vi "测验程序3.vi"() -> ()   [LabVIEW 2017]
uses:
  <vilib>/userdefined/High Color/IMAQdx.ctl
  <vilib>/Platform/TimedLoop/XDataNode/timing_clust.ctl
  <vilib>/Platform/TimedLoop/XDataNode/nitl_modes.ctl
  <vilib>/Platform/TimedLoop/XDataNode/wakeup.ctl
  <vilib>/myRIO/Common/Instrument Driver Framework/myRIO v1.0/UART/vis/myRIO v1.0 Close UART.vi
  <vilib>/FPGAPlugInAG/myRIO-1900/niLvFpga_Open_myRIO-1900.vi
  <vilib>/rvi/interface/common/dynamic/niFpgaDynamicAddResources.vi
  <vilib>/myRIO/Common/Instrument Driver Framework/Utilities/vis/FPGA Ref Manager.vi
  <vilib>/Utility/error.llb/Error Cluster From Error Code.vi
  <vilib>/myRIO/Common/Instrument Driver Framework/Utilities/vis/Ref Counter.vi
  <vilib>/rvi/errors/niLvFpgaAdjustHostInterfaceError.vi
  <vilib>/FPGAPlugInAG/Dynamic/niLvFpga_Close_Dynamic.vi
  <vilib>/myRIO/Common/Instrument Driver Framework/myRIO v1.0/myRIO v1.0 Reset FPGA.vi
  <vilib>/myRIO/Common/Instrument Driver Framework/myRIO v1.0/IRQ/vis/myRIO v1.0 IRQ Info FGV.vi
  <vilib>/myRIO/Common/Instrument Driver Framework/myRIO v1.0/IRQ/vis/myRIO v1.0 Timer IRQ Info FGV.vi
  <vilib>/myRIO/Common/Instrument Driver Framework/myRIO v1.0/IRQ/vis/myRIO v1.0 ISR Agent.vi
  <vilib>/Platform/TimedLoop/XDataNode/XDataNode.xnode
  <vilib>/rvi/interface/nirviOpenFPGA/nirviOpenFPGA.xnode
  <vilib>/rvi/interface/nirviReadWriteControl/nirviReadWriteControl.xnode
  <vilib>/rvi/interface/nirviCloseFPGA/nirviCloseFPGA.xnode
  <vilib>/Platform/TimedLoop/XDataNode/XDNodeRunTimeDep.lvlib
  <vilib>/myRIO/Instrument Drivers/Utilities/Utilities.lvlib
  NiFpgaLv.dll
  <vilib>/rvi/interface/Simulation/niFpgaSimulationCallBeginRW.vi
  <vilib>/vision/driver/NI_Vision_Acquisition_Software.lvlib
  <vilib>/vision/NI_Vision_Development_Module.lvlib
panel:
  out "货物类型":u32
  in  "Reset":bool
  in  "Reset to gait 0":bool
  in  "停止":bool
  out "数量":i32[](array[numeric])
  in  "保留图像？":bool
  in  "停止 2":bool
  in  "初始步态":u16
  in  "开始":bool
  out "QTI":bool
  out "当前步态":u16
  out "超声波":u32[](array[numeric])
  # "4小蓝"
  # "3小红"
  # "2大蓝"
  # "100000"
  # "1大红"
  # "70000"
  # "0异常"
  # "25000"
  # "14600夹取高度"
  # "700夹住"
  # "-1010"
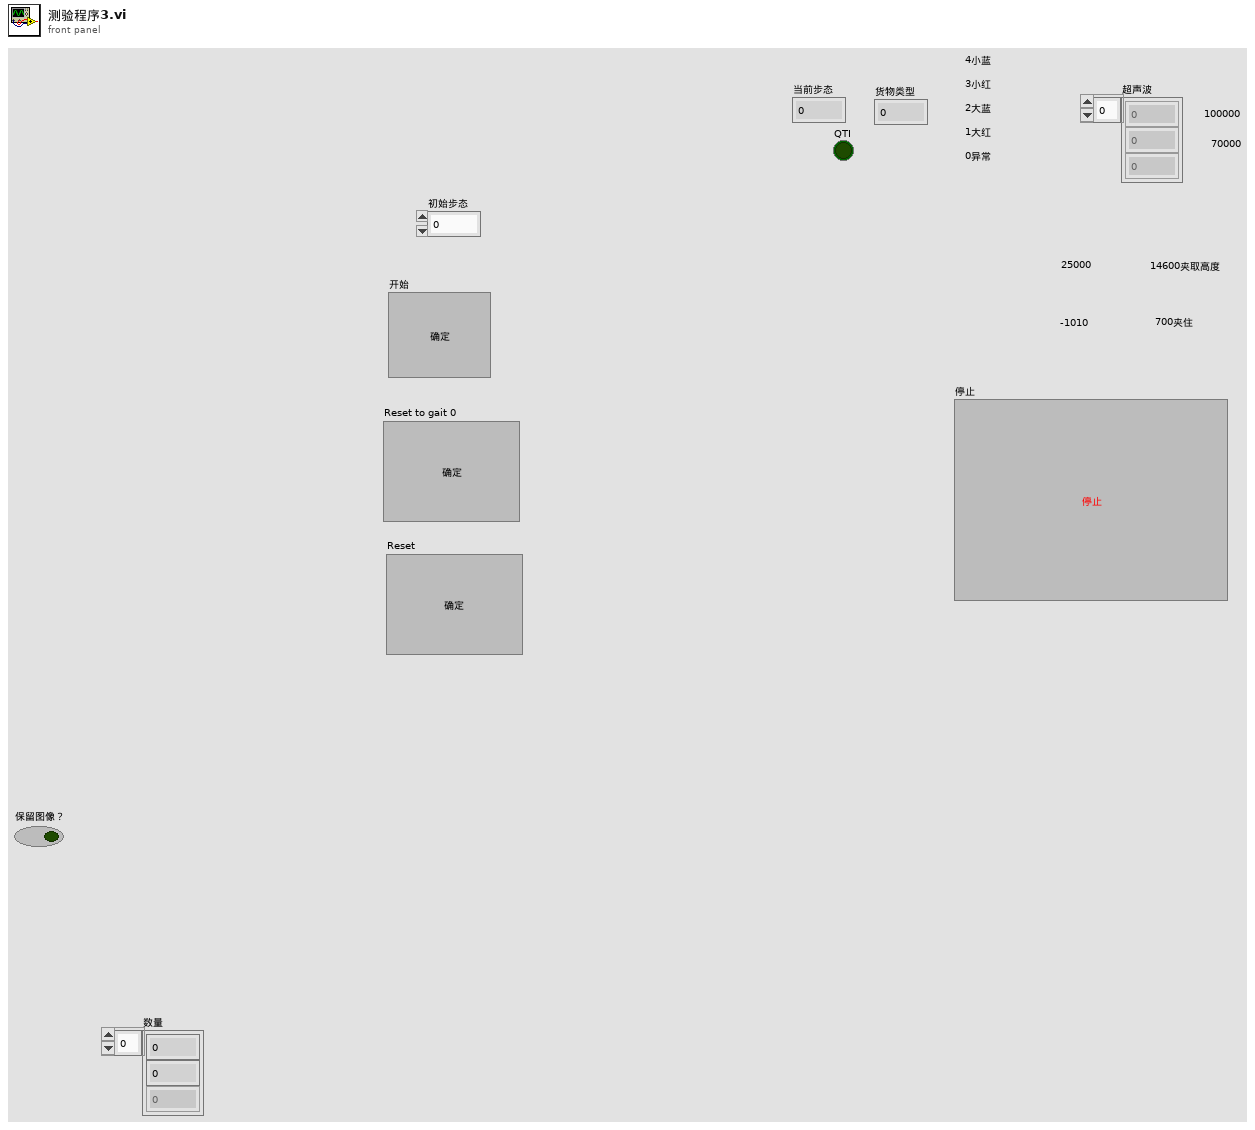
[diagram p1: front panel]
types:
  T1 = typedef "IMAQdx.ctl" = refnum<k21>
  T2 = typedef "IMAQ Image.ctl" = refnum<image>
  T3 = typedef "XDNodeRunTimeDep.lvlib/timing_clust.ctl" = cluster{"Expected End [f-1]":u64, "Actual End [f-1]":u64, "Finished Late? [f-1]":bool, "Expected End [i-1]":u64, "Actual End [i-1]":u64, "Finished Late? [i-1]":bool, "Expected Start [i]":u64, "Actual Start [i]":u64, "Expected Start [f]":u64, "Actual Start [f]":u64, "Source Name":string, "Structure Name":string, "Period":i64, "Deadline":i64, "Offset":i64, "Start":i64, "Priority":i32, "Timeout":i32, "Mode":T4, "Wakeup Reason":T5, "Error":errorcluster, "Source Type":string, "Secondary Source Type":string, "Global End Time":u64, "Global Start Time":u64, "Frame Duration":u64, "Iteration Duration":u64, "Assigned CPU":i32, "I/O Scan Engine Mode":u32}
  T4 = typedef "XDNodeRunTimeDep.lvlib/nitl_modes.ctl" = enum32{"No Change", "Process missed periods, maintain original phase", "Discard missed periods, maintain original phase", "Process missed periods, ignore original phase", "Discard missed periods, ignore original phase"}
  T5 = typedef "XDNodeRunTimeDep.lvlib/wakeup.ctl" = enum32{"Normal", "Aborted", "Asynchronous wakeup", "Timing source error", "Timed loop error", "Timeout"}
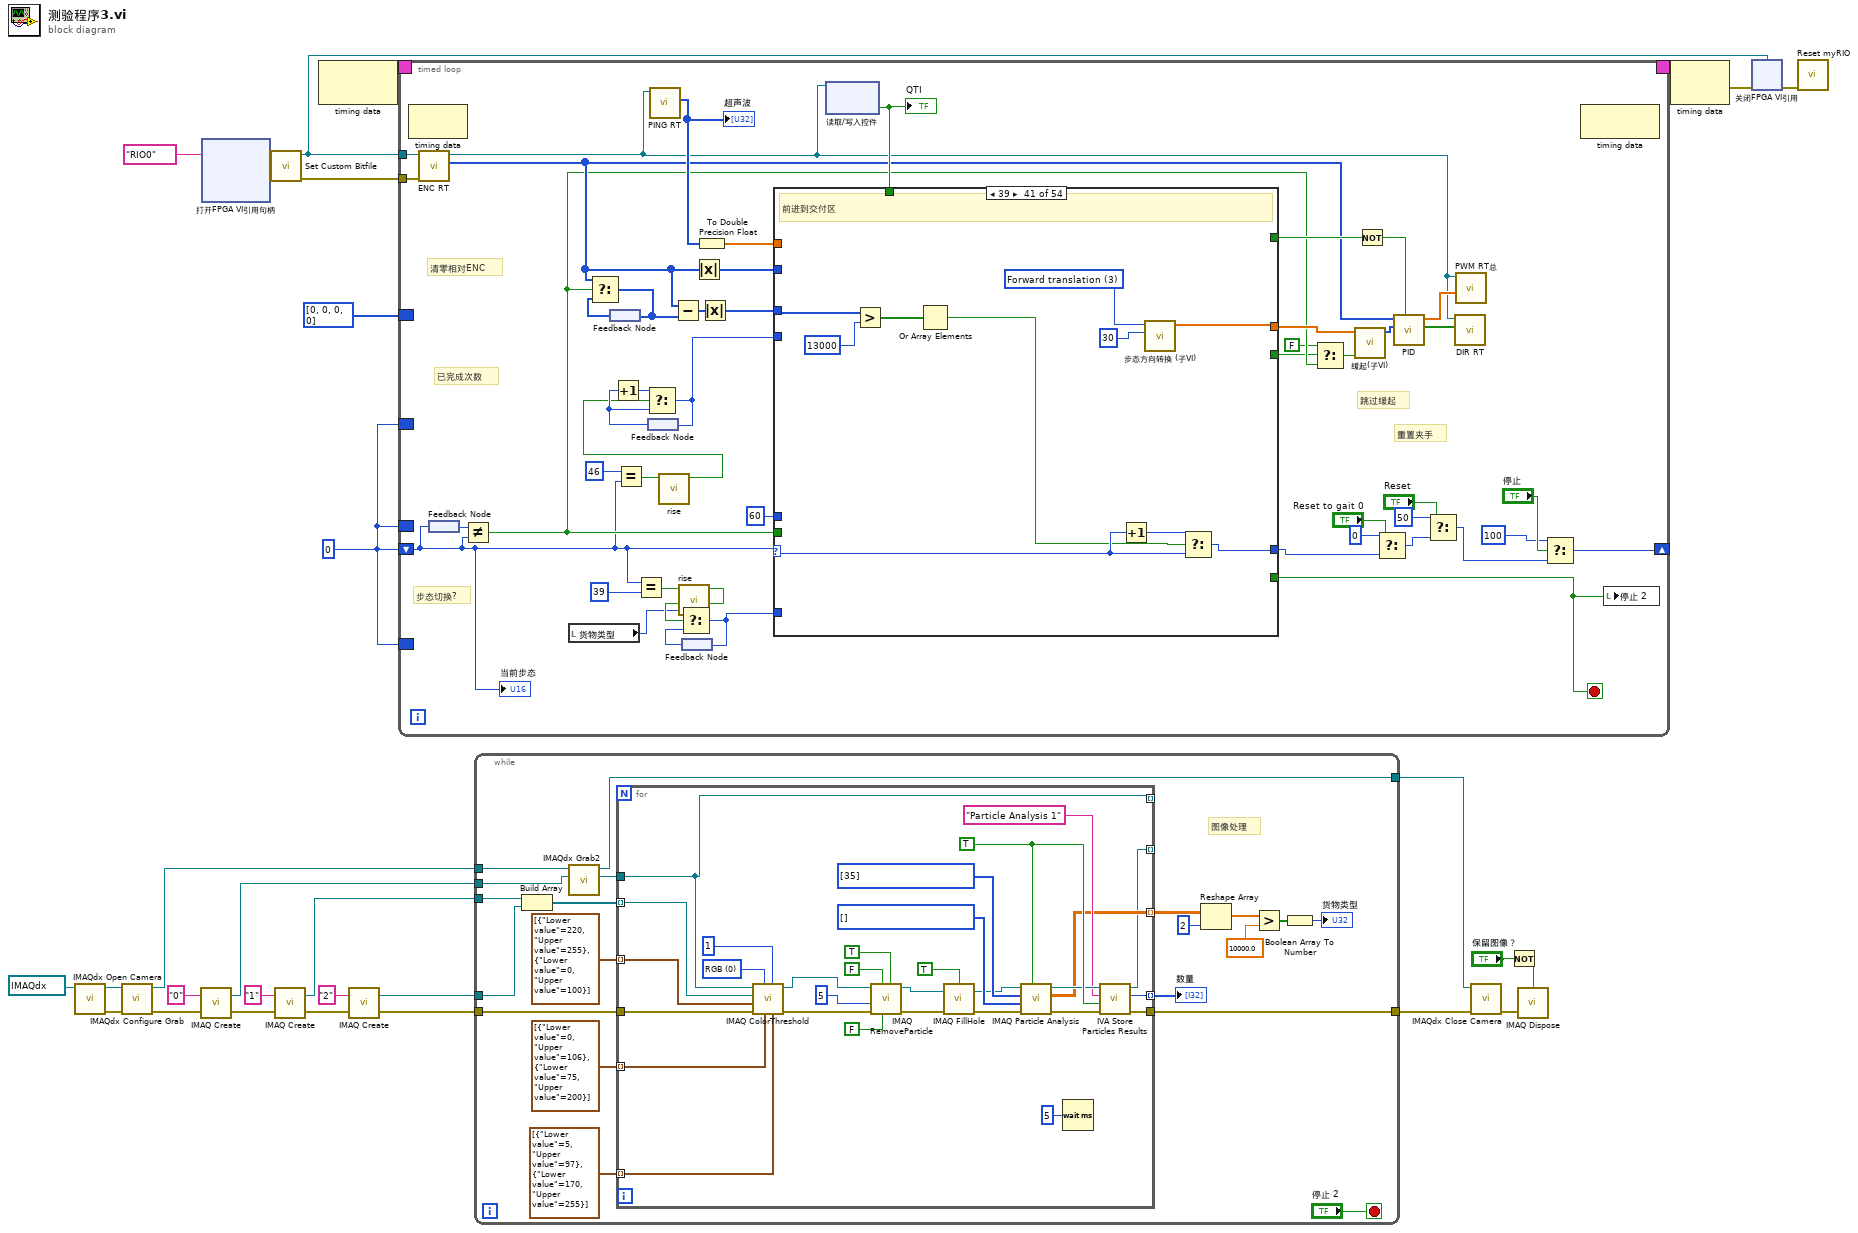
[diagram p0: block diagram]
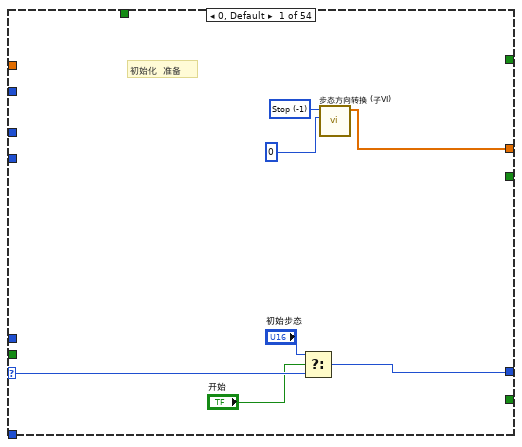
[diagram p2: hidden frame]
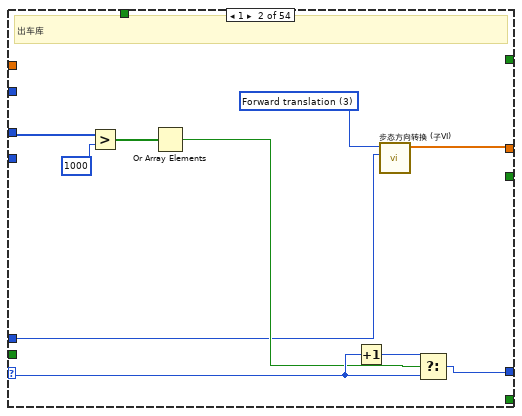
[diagram p3: hidden frame]
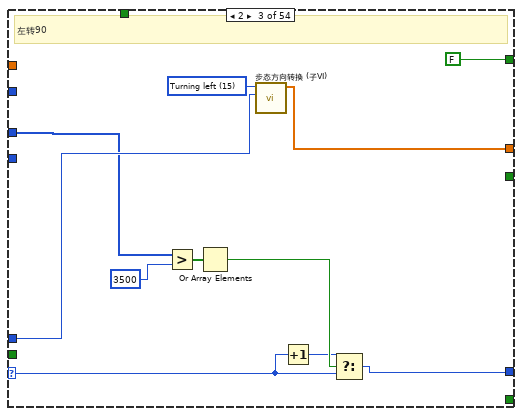
[diagram p4: hidden frame]
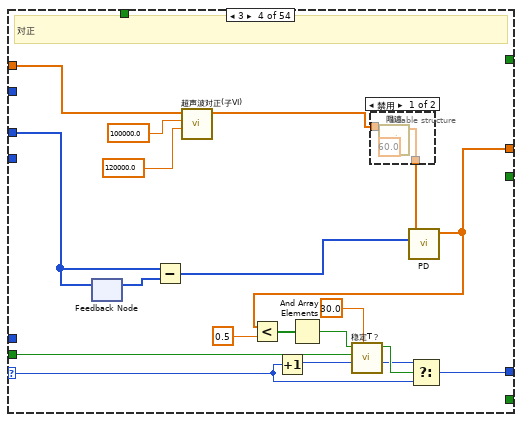
[diagram p5: hidden frame]
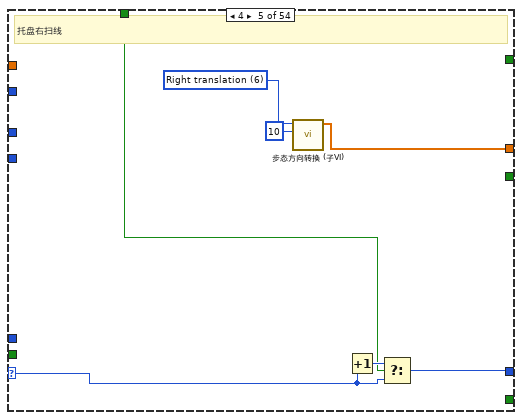
[diagram p7: hidden frame]
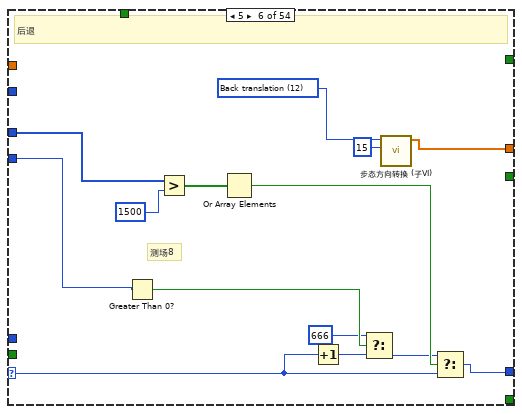
[diagram p8: hidden frame]
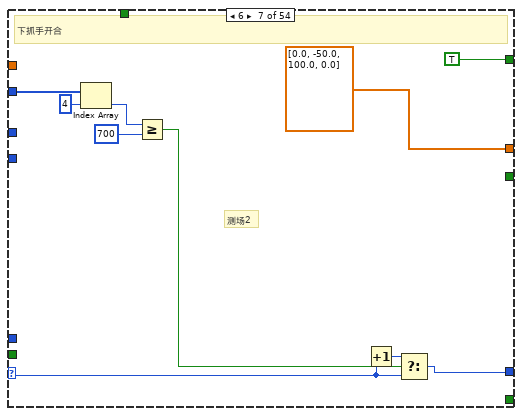
[diagram p9: hidden frame]
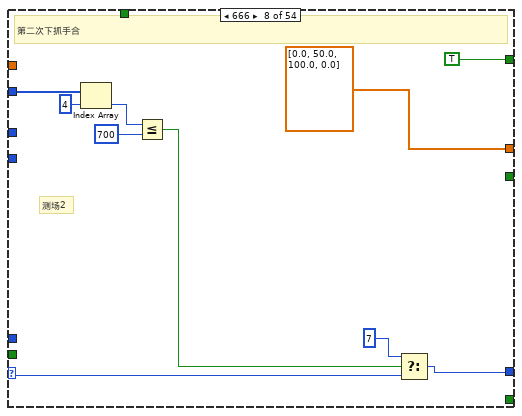
[diagram p10: hidden frame]
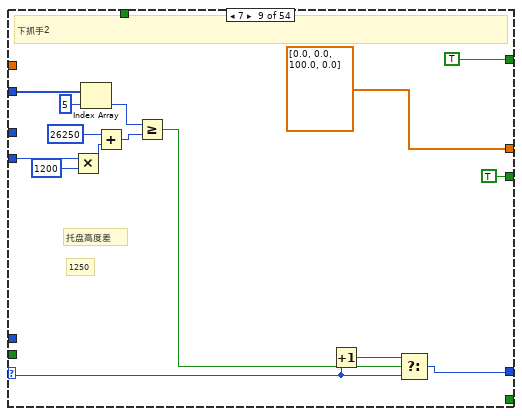
[diagram p11: hidden frame]
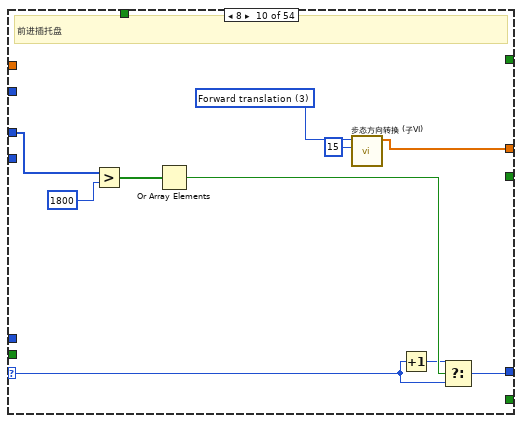
[diagram p12: hidden frame]
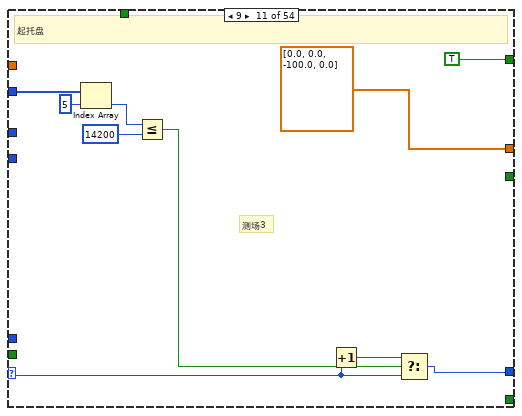
[diagram p13: hidden frame]
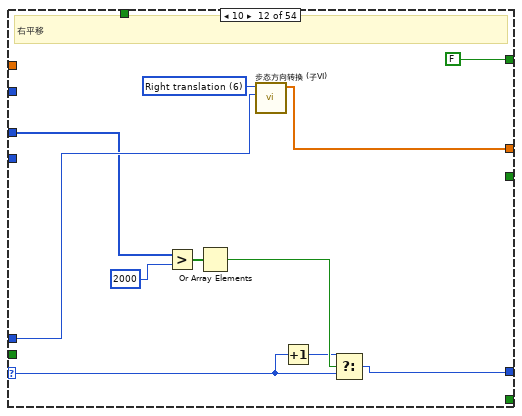
[diagram p14: hidden frame]
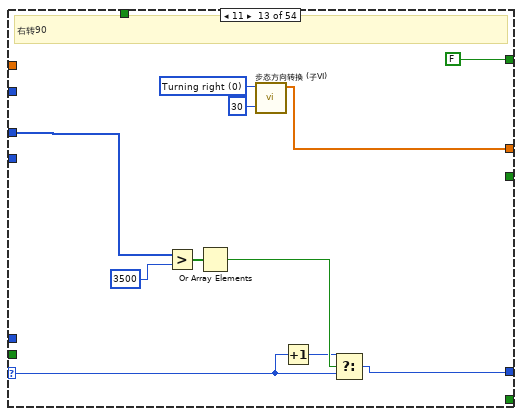
[diagram p15: hidden frame]
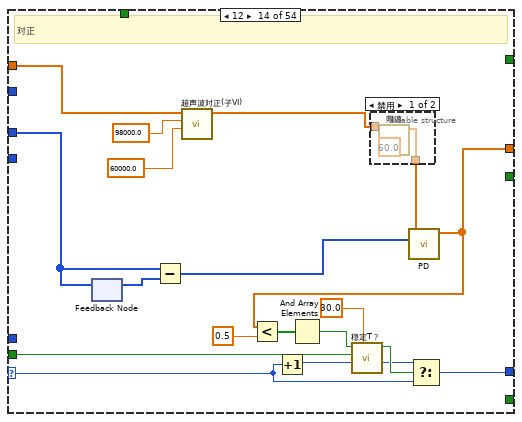
[diagram p16: hidden frame]
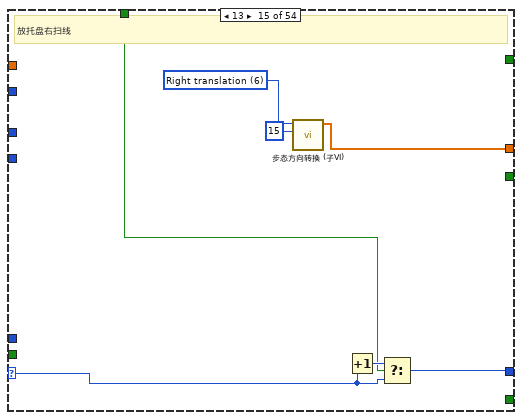
[diagram p18: hidden frame]
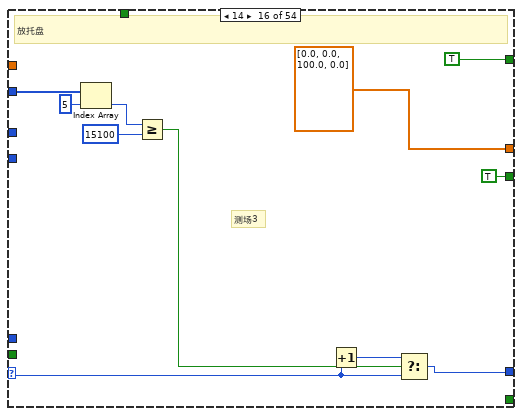
[diagram p19: hidden frame]
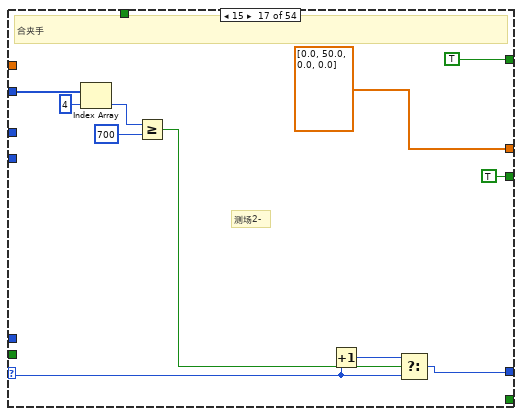
[diagram p20: hidden frame]
diagram:
  w1 = u16 0 ("初始步态")
  n1 = call <vilib>:"IMAQdx Open Camera.vi"("Session In"=T1 "cam0") -> ("error out"=w16:errorcluster, "Session Out"=w15:T1)  [unwired: 9 in]
  n2 = call <vilib>:"IMAQdx Configure Grab.vi"("error in"=w16, "Session In"=w15) -> ("error out"=w13:errorcluster, "Session Out"=w20:T1)  [unwired: 8 in]
  n3 = call "IMAQ Create"("Image Name"="0", "error in (no error)"=w13) -> ("New Image"=w18:T2, "error out"=w11:errorcluster)  [unwired: 3 in]
  n4 = xnode "打开FPGA VI引用句柄"("资源名称"=tag "RIO0") -> ("FPGA VI引用输出"=w25:refnum<k20>, "错误输出"=w24:errorcluster)  [unwired: 1 in]
  n5 = call <vilib>:"Set Custom Bitfile.vi"("error in (no error)"=w24, "Custom FPGA Reference In"=w25) -> ("error out"=w23:errorcluster, "Custom FPGA Reference Out"=w21:refnum<k20>)  [unwired: 8 in]
  n6 = call "IMAQ Create"("Image Name"="1", "error in (no error)"=w11) -> ("New Image"=w8:T2, "error out"=w9:errorcluster)  [unwired: 3 in]
  n7 = node-c288() -> (w30:T3)  [unwired: 1 in]
  n8 = call "IMAQ Create"("Image Name"="2", "error in (no error)"=w9) -> ("New Image"=w7:T2, "error out"=w6:errorcluster)  [unwired: 3 in]
  n9 = timed-loop {
    timing: w30 -> [_]
    timing-out: [_] -> w29
    shift-right: [w58] -> _
    shift-left: w1 -> [w33]
    border: w1 -> [_]
    border: i32[] [0, 0, 0, 0] ("ENC") -> [_]
    tunnel: w23 -> [w75]
    tunnel: w21 -> [w72]
    border: w1 -> [_]
    border: w1 -> [_]
    stop <- w44 stop-if-true
    # "已完成次数"
    # "重置夹手"
    # "跳过缓起"
    # "步态切换?"
    # "清零相对ENC"
    n10 = node-c288() -> ()  [unwired: 1 in, 1 out]
    n11 = call "ENC RT.vi"("错误输入（无错误）"=w75, "Custom FPGA Reference Out"=w72) -> ("ENC"=w62:i32[], "FPGA VI引用输出"=w60:refnum<k20>)  [unwired: 7 in, 1 out]
    n12 = feedback-in #1(w33) -> ()
    n13 = feedback #1() -> (w76:u16)
    n14 = Not Equal?(x=w76, y=w33) -> (x != y?=w52:bool)
    n15 = local read "货物类型"() -> (w32:u32)
    n16 = feedback #2() -> (w74:i32[])
    n17 = Select(t=w62, s=w52, f=w74) -> (s? t:f=w59:i32[])
    n18 = feedback-in #2(w59) -> ()
    n19 = Equal?(x=u16 46 ("y"), y=w33) -> (x = y?=w39:bool)
    n20 = Equal?(x=w33, y=u16 39) -> (x = y?=w36:bool)
    n21 = feedback #3() -> (w42:u16)
    n22 = Increment(x=w42) -> (x+1=w41:u16)
    n23 = call "PING RT.vi"("引用句柄输入"=w60) -> ("PING"=w66:u32[])  [unwired: 8 in, 2 out]
    "超声波" <- w66
    n24 = call "rise.vi"("TF"=w39) -> ("UP?"=w38:bool)  [unwired: 10 in]
    n25 = Select(t=w41, s=w38, f=w42) -> (s? t:f=w40:u16)
    n26 = feedback-in #3(w40) -> ()
    n27 = Subtract(x=w62, y=w59) -> (x-y=w67:i32[])
    n28 = call "rise.vi"("TF"=w36) -> ("UP?"=w37:bool)  [unwired: 10 in]
    n29 = feedback #4() -> (w35:u32)
    n30 = Select(t=w32, s=w37, f=w35) -> (s? t:f=w31:u32)
    n31 = feedback-in #4(w31) -> ()
    n32 = Absolute Value(x=w62) -> (abs(x)=w61:i32[])
    n33 = To Double Precision Float(number=w66) -> (double precision float=w65:dbl[])
    n34 = Absolute Value(x=w67) -> (abs(x)=w63:i32[])
    n35 = xnode "读取/写入控件"("FPGA VI引用输入"=w60) -> ("QTI"=w64:bool)  [unwired: 1 in, 2 out]
    "QTI" <- w64
    n36 = case shown="39" w33 {
      selector: w33 -> [w84 w88 w99 w122 w132 w145 w156 w167 w182 w186 w202 w208 w220 w242 w252 w264 w275 w279 w292 w325 w336 w347 w354 w378 w384 w395 w405 w415 w421 w455 w461 w469 w491 w497 w508 w516 w529 w533 w549 w556 w565 w588 w602 w614 w622 w637 w643 w666 w679 w691 w702 w710 w718 w730]
      tunnel: [w79 w95 w100 w116 w133 w147 dbl[] [0.0, -50.0, 100.0, 0.0] ("输出") dbl[] [0.0, 50.0, 100.0, 0.0] ("输出") dbl[] [0.0, 0.0, 100.0, 0.0] ("输出") w192 dbl[] [0.0, 0.0, -100.0, 0.0] ("输出") w209 w221 w236 w253 dbl[] [0.0, 0.0, 100.0, 0.0] ("输出") dbl[] [0.0, 50.0, 0.0, 0.0] ("输出") w281 w293 w313 w337 dbl[] [0.0, 0.0, -100.0, 0.0] ("输出") w355 w365 w385 dbl[] [0.0, 0.0, 50.0, 0.0] ("输出") dbl[] [0.0, 10.0, 0.0, 0.0] ("输出") dbl[] [0.0, 0.0, -50.0, 0.0] ("输出") w422 w443 w462 w470 w479 w498 dbl[] [0.0, -10.0, 0.0, 0.0] ("输出") w518 dbl[] [0.0, 0.0, 100.0, 0.0] ("输出") w539 dbl[] [0.0, 0.0, -100.0, 0.0] ("输出") w557 w572 w582 w603 dbl[] [0.0, 2.0, 100.0, 0.0] ("输出") w624 w627 w644 w660 dbl[] [0.0, 50.0, -100.0, 0.0] ("输出") dbl[] [0.0, 0.0, -100.0, 0.0] ("输出") w700 dbl[] [0.0, 10.0, 0.0, 0.0] ("输出") dbl[] [0.0, 0.0, 0.0, 0.0] ("输出") dbl[] [0.0, 0.0, 0.0, 0.0] ("输出")] -> w71
      tunnel: 60 ("思币得") -> [_ w86 w101 _ _ _ _ _ _ _ _ w210 _ _ _ _ _ _ _ _ _ _ _ _ _ _ _ _ w423 _ _ _ _ _ _ _ _ _ _ _ _ _ _ _ _ _ w645 _ _ _ w694 _ _ _]
      tunnel: [w82 w91 w106 w121 w130 w146 w158 w168 w183 w185 w203 w215 w226 w241 w250 w265 w276 w280 w298 w327 w334 w348 w360 w380 w382 w396 w406 w416 w428 w457 w459 w475 w493 w495 w509 w517 w530 w532 w550 w562 w568 w587 w600 w615 w623 w638 w650 w665 w681 w692 w703 w712 w720 w730] -> w55
      tunnel: [_ _ FALSE ("继电器") _ _ _ TRUE ("继电器") TRUE ("继电器") TRUE ("继电器") _ TRUE ("继电器") FALSE ("继电器") FALSE ("继电器") _ _ TRUE ("继电器") TRUE ("继电器") _ FALSE ("继电器") FALSE ("继电器") _ TRUE ("继电器") FALSE ("继电器") FALSE ("继电器") _ TRUE ("继电器") TRUE ("继电器") TRUE ("继电器") FALSE ("继电器") FALSE ("继电器") _ FALSE ("继电器") FALSE ("继电器") _ TRUE ("继电器") _ TRUE ("继电器") _ TRUE ("继电器") FALSE ("继电器") _ _ _ TRUE ("继电器") _ _ FALSE ("继电器") _ TRUE ("继电器") TRUE ("继电器") _ TRUE ("继电器") _ _] -> w69
      tunnel: w63 -> [_ w93 w97 w119 _ w141 _ _ _ w189 _ w206 w218 w239 _ _ _ w282 w290 w319 _ _ w352 w371 _ _ _ _ w419 w449 _ w467 w485 _ _ w512 _ w536 _ w554 w570 w585 _ _ w618 w633 w641 w663 _ _ w696 _ _ _]
      tunnel: w65 -> [_ _ _ w124 _ _ _ _ _ _ _ _ _ w244 _ _ _ _ _ w323 _ _ _ w376 _ _ _ _ _ w453 _ _ w489 _ _ _ _ _ _ _ _ w590 _ _ _ _ _ w668 _ _ _ _ _ _]
      tunnel: w52 -> [_ _ _ w111 _ _ _ _ _ _ _ _ _ w231 _ _ _ _ _ w312 w331 _ _ w364 _ _ _ _ _ w442 _ _ w478 _ _ _ _ _ _ _ _ w577 w598 _ _ _ _ w655 _ _ _ _ _ _]
      tunnel: w64 -> [_ _ _ _ w129 _ _ _ _ _ _ _ _ _ w249 _ _ _ _ _ w329 _ _ _ w381 _ _ _ _ _ w458 _ _ w494 _ _ _ _ _ _ _ _ w596 _ _ _ _ _ _ _ _ _ _ _]
      tunnel: w61 -> [_ _ _ _ _ _ w150 w161 w176 _ w196 _ _ _ _ w258 w269 _ _ _ _ w341 _ _ _ w389 w399 w409 _ _ _ _ _ _ w502 _ w523 _ w543 _ _ _ _ w608 _ _ _ _ w673 w685 _ w704 _ _]
      tunnel: [_ _ _ _ _ _ _ _ _ _ _ _ _ _ _ _ _ _ _ _ _ _ _ _ _ _ _ _ _ _ _ _ _ _ _ _ _ _ _ _ _ _ _ _ _ _ _ _ _ _ _ _ _ TRUE ("停止 2")] -> w44
      tunnel: [_ _ _ _ _ _ _ _ TRUE ("t") _ _ _ _ _ _ TRUE ("t") TRUE ("t") _ _ _ _ _ _ _ _ _ _ _ _ _ _ _ _ _ _ _ TRUE ("t") _ _ _ _ _ _ TRUE ("t") _ _ _ _ _ TRUE ("t") _ _ _ _] -> w49
      tunnel: w31 -> [_ _ _ _ _ _ _ _ _ _ _ _ _ _ _ _ _ _ _ _ _ _ _ _ _ _ _ _ _ _ _ _ _ _ _ _ _ _ _ _ _ _ w597 _ _ _ _ _ _ _ _ _ _ _]
      tunnel: w40 -> [_ _ _ _ _ w138 _ _ w172 _ _ _ _ _ _ _ _ _ _ _ w332 _ _ _ _ _ _ _ _ _ _ _ _ _ _ _ _ _ _ _ _ _ _ _ _ _ _ _ _ _ _ _ _ _]
      frame 0, Default {
        w85 = i8 -1 items=["Stop"=-1, "Right translation"=6, "Back translation"=12, "Turning right"=0, "Turning left"=15, "Forward translation"=3, "Left translation"=9, "Gyro rotating"=16] ("Gait")
        # "初始化  准备"
        n37 = Select(t="初始步态", s="开始", f=w84) -> (s? t:f=w82:u16)
        n38 = call "步态方向转换 (子VI).vi"("速度"=0 ("长度"), "Gait"=w85) -> ("输出"=w79:dbl[])  [unwired: 9 in]
      }
      frame 1 {
        w94 = i8 3 items=["Stop"=-1, "Right translation"=6, "Back translation"=12, "Turning right"=0, "Turning left"=15, "Forward translation"=3, "Left translation"=9, "Gyro rotating"=16] ("Gait")
        # "出车库"
        n39 = Greater?(x=w93, y=1000) -> (0:w90:bool[])
        n40 = Or Array Elements(Boolean array=w90) -> (logical OR=w87:bool)
        n41 = Increment(x=w88) -> (x+1=w89:u16)
        n42 = call "步态方向转换 (子VI).vi"("速度"=w86, "Gait"=w94) -> ("输出"=w95:dbl[])  [unwired: 9 in]
        n43 = Select(t=w89, s=w87, f=w88) -> (s? t:f=w91:u16)
      }
      frame 2 {
        w102 = i8 15 items=["Stop"=-1, "Right translation"=6, "Back translation"=12, "Turning right"=0, "Turning left"=15, "Forward translation"=3, "Left translation"=9, "Gyro rotating"=16] ("Gait")
        # "左转90"
        n44 = Greater?(x=w97, y=3500 ("次数")) -> (0:w104:bool[])
        n45 = Or Array Elements(Boolean array=w104) -> (logical OR=w103:bool)
        n46 = call "步态方向转换 (子VI).vi"("速度"=w101, "Gait"=w102) -> ("输出"=w100:dbl[])  [unwired: 9 in]
        n47 = Increment(x=w99) -> (x+1=w98:u16)
        n48 = Select(t=w98, s=w103, f=w99) -> (s? t:f=w106:u16)
      }
      frame 3 {
        # "对正"
        n49 = feedback-in #5(w119) -> ()
        n50 = feedback #5() -> (w118:i32[])  [unwired: 1 in]
        n51 = Subtract(x=w119, y=w118) -> (x-y=w117:i32[])
        n52 = call "超声波对正(子VI).vi"("LFT"=120000.0, "FWD"=100000.0, "超声波"=w124) -> ("数组输出"=w123:dbl[])  [unwired: 8 in]
        n53 = Increment(x=w122) -> (x+1=w107:u16)
        n54 = disable-structure shown="禁用" {
          disable-tunnel: w123 -> [w127 w128]
          disable-tunnel: [w125 w128] -> w120
          frame Disabled {
            n55 = call "限速.vi"("最大值"=60.0, "输入"=w127) -> ("数组"=w125:dbl[])  [unwired: 9 in]
          }
          frame Enabled {
          }
        }
        n56 = call "PD.vi"("ENC"=w117, "SET"=w120) -> ("output"=w116:dbl[])  [unwired: 9 in]
        n57 = Less?(x=w116, y=0.5) -> (x < y?=w114:bool[])
        n58 = And Array Elements(Boolean array=w114) -> (logical AND=w113:bool)
        n59 = call "稳定T？.vi"("次数(100)"=30.0, "Reset"=w111, "输入"=w113) -> ("TT？"=w112:bool)  [unwired: 8 in]
        n60 = Select(t=w107, s=w112, f=w122) -> (s? t:f=w121:u16)
      }
      frame 4 {
        w135 = i8 6 items=["Stop"=-1, "Right translation"=6, "Back translation"=12, "Turning right"=0, "Turning left"=15, "Forward translation"=3, "Left translation"=9, "Gyro rotating"=16] ("Gait")
        # "托盘右扫线"
        n61 = call "步态方向转换 (子VI).vi"("速度"=10, "Gait"=w135) -> ("输出"=w133:dbl[])  [unwired: 9 in]
        n62 = Increment(x=w132) -> (x+1=w131:u16)
        n63 = Select(t=w131, s=w129, f=w132) -> (s? t:f=w130:u16)
      }
      frame 5 {
        w149 = i8 12 items=["Stop"=-1, "Right translation"=6, "Back translation"=12, "Turning right"=0, "Turning left"=15, "Forward translation"=3, "Left translation"=9, "Gyro rotating"=16] ("Gait")
        # "测场8"
        # "后退"
        n64 = Greater Than 0?(x=w138) -> (x > 0?=w137:bool)
        n65 = Greater?(x=w141, y=1500) -> (0:w142:bool[])
        n66 = Or Array Elements(Boolean array=w142) -> (logical OR=w140:bool)
        n67 = Increment(x=w145) -> (x+1=w144:u16)
        n68 = Select(t=u16 666 ("f"), s=w137, f=w144) -> (s? t:f=w139:u16)
        n69 = call "步态方向转换 (子VI).vi"("速度"=15, "Gait"=w149) -> ("输出"=w147:dbl[])  [unwired: 9 in]
        n70 = Select(t=w139, s=w140, f=w145) -> (s? t:f=w146:u16)
      }
      frame 6 {
        # "测场2"
        # "下抓手开合"
        n71 = Index Array(array=w150, index=4 ("索引")) -> (element=w153:i32)
        n72 = Greater Or Equal?(x=w153, y=700) -> (x >= y?=w151:bool)
        n73 = Increment(x=w156) -> (x+1=w157:u16)
        n74 = Select(t=w157, s=w151, f=w156) -> (s? t:f=w158:u16)
      }
      frame 666 {
        # "测场2"
        # "第二次下抓手合"
        n75 = Index Array(array=w161, index=4 ("索引")) -> (element=w164:i32)
        n76 = Less Or Equal?(x=w164, y=700) -> (x <= y?=w162:bool)
        n77 = Select(t=u16 7, s=w162, f=w167) -> (s? t:f=w168:u16)
      }
      frame 7 {
        # "1250"
        # "托盘高度差"
        # "下抓手2"
        n78 = Multiply(x=w172, y=u16 1200) -> (x*y=w173:u16)
        n79 = Index Array(array=w176, index=5 ("索引")) -> (element=w179:i32)
        n80 = Add(x=26250 ("y"), y=w173) -> (x+y=w174:i32)
        n81 = Greater Or Equal?(x=w179, y=w174) -> (x >= y?=w177:bool)
        n82 = Increment(x=w182) -> (x+1=w170:u16)
        n83 = Select(t=w170, s=w177, f=w182) -> (s? t:f=w183:u16)
      }
      frame 8 {
        w194 = i8 3 items=["Stop"=-1, "Right translation"=6, "Back translation"=12, "Turning right"=0, "Turning left"=15, "Forward translation"=3, "Left translation"=9, "Gyro rotating"=16] ("Gait")
        # "前进插托盘"
        n84 = Greater?(x=w189, y=1800) -> (0:w190:bool[])
        n85 = Or Array Elements(Boolean array=w190) -> (logical OR=w188:bool)
        n86 = call "步态方向转换 (子VI).vi"("速度"=15, "Gait"=w194) -> ("输出"=w192:dbl[])  [unwired: 9 in]
        n87 = Increment(x=w186) -> (x+1=w187:u16)
        n88 = Select(t=w187, s=w188, f=w186) -> (s? t:f=w185:u16)
      }
      frame 9 {
        # "测场3"
        # "起托盘"
        n89 = Index Array(array=w196, index=5 ("索引")) -> (element=w199:i32)
        n90 = Less Or Equal?(x=w199, y=14200) -> (x <= y?=w197:bool)
        n91 = Increment(x=w202) -> (x+1=w195:u16)
        n92 = Select(t=w195, s=w197, f=w202) -> (s? t:f=w203:u16)
      }
      frame 10 {
        w211 = i8 6 items=["Stop"=-1, "Right translation"=6, "Back translation"=12, "Turning right"=0, "Turning left"=15, "Forward translation"=3, "Left translation"=9, "Gyro rotating"=16] ("Gait")
        # "右平移"
        n93 = Greater?(x=w206, y=2000 ("次数")) -> (0:w213:bool[])
        n94 = Or Array Elements(Boolean array=w213) -> (logical OR=w212:bool)
        n95 = call "步态方向转换 (子VI).vi"("速度"=w210, "Gait"=w211) -> ("输出"=w209:dbl[])  [unwired: 9 in]
        n96 = Increment(x=w208) -> (x+1=w207:u16)
        n97 = Select(t=w207, s=w212, f=w208) -> (s? t:f=w215:u16)
      }
      frame 11 {
        w222 = i8 0 items=["Stop"=-1, "Right translation"=6, "Back translation"=12, "Turning right"=0, "Turning left"=15, "Forward translation"=3, "Left translation"=9, "Gyro rotating"=16] ("Gait")
        # "右转90"
        n98 = Greater?(x=w218, y=3500 ("次数")) -> (0:w224:bool[])
        n99 = Or Array Elements(Boolean array=w224) -> (logical OR=w223:bool)
        n100 = call "步态方向转换 (子VI).vi"("速度"=30, "Gait"=w222) -> ("输出"=w221:dbl[])  [unwired: 9 in]
        n101 = Increment(x=w220) -> (x+1=w219:u16)
        n102 = Select(t=w219, s=w223, f=w220) -> (s? t:f=w226:u16)
      }
      frame 12 {
        # "对正"
        n103 = feedback-in #6(w239) -> ()
        n104 = feedback #6() -> (w238:i32[])  [unwired: 1 in]
        n105 = Subtract(x=w239, y=w238) -> (x-y=w237:i32[])
        n106 = call "超声波对正(子VI).vi"("LFT"=60000.0, "FWD"=98000.0, "超声波"=w244) -> ("数组输出"=w243:dbl[])  [unwired: 8 in]
        n107 = Increment(x=w242) -> (x+1=w227:u16)
        n108 = disable-structure shown="禁用" {
          disable-tunnel: w243 -> [w247 w248]
          disable-tunnel: [w245 w248] -> w240
          frame Disabled {
            n109 = call "限速.vi"("最大值"=60.0, "输入"=w247) -> ("数组"=w245:dbl[])  [unwired: 9 in]
          }
          frame Enabled {
          }
        }
        n110 = call "PD.vi"("ENC"=w237, "SET"=w240) -> ("output"=w236:dbl[])  [unwired: 9 in]
        n111 = Less?(x=w236, y=0.5) -> (x < y?=w234:bool[])
        n112 = And Array Elements(Boolean array=w234) -> (logical AND=w233:bool)
        n113 = call "稳定T？.vi"("次数(100)"=30.0, "Reset"=w231, "输入"=w233) -> ("TT？"=w232:bool)  [unwired: 8 in]
        n114 = Select(t=w227, s=w232, f=w242) -> (s? t:f=w241:u16)
      }
      frame 13 {
        w255 = i8 6 items=["Stop"=-1, "Right translation"=6, "Back translation"=12, "Turning right"=0, "Turning left"=15, "Forward translation"=3, "Left translation"=9, "Gyro rotating"=16] ("Gait")
        # "放托盘右扫线"
        n115 = call "步态方向转换 (子VI).vi"("速度"=15, "Gait"=w255) -> ("输出"=w253:dbl[])  [unwired: 9 in]
        n116 = Increment(x=w252) -> (x+1=w251:u16)
        n117 = Select(t=w251, s=w249, f=w252) -> (s? t:f=w250:u16)
      }
      frame 14 {
        # "测场3"
        # "放托盘"
        n118 = Index Array(array=w258, index=5 ("索引")) -> (element=w261:i32)
        n119 = Greater Or Equal?(x=w261, y=15100) -> (x >= y?=w259:bool)
        n120 = Increment(x=w264) -> (x+1=w257:u16)
        n121 = Select(t=w257, s=w259, f=w264) -> (s? t:f=w265:u16)
      }
      frame 15 {
        # "测场2-"
        # "合夹手"
        n122 = Index Array(array=w269, index=4 ("索引")) -> (element=w272:i32)
        n123 = Greater Or Equal?(x=w272, y=700) -> (x >= y?=w270:bool)
        n124 = Increment(x=w275) -> (x+1=w267:u16)
        n125 = Select(t=w267, s=w270, f=w275) -> (s? t:f=w276:u16)
      }
      frame 16 {
        w287 = i8 12 items=["Stop"=-1, "Right translation"=6, "Back translation"=12, "Turning right"=0, "Turning left"=15, "Forward translation"=3, "Left translation"=9, "Gyro rotating"=16] ("Gait")
        # "测场4"
        # "后退出组装架"
        n126 = Greater?(x=w282, y=2000) -> (0:w284:bool[])
        n127 = Or Array Elements(Boolean array=w284) -> (logical OR=w283:bool)
        n128 = Increment(x=w279) -> (x+1=w278:u16)
        n129 = call "步态方向转换 (子VI).vi"("速度"=30, "Gait"=w287) -> ("输出"=w281:dbl[])  [unwired: 9 in]
        n130 = Select(t=w278, s=w283, f=w279) -> (s? t:f=w280:u16)
      }
      frame 17 {
        w294 = i8 15 items=["Stop"=-1, "Right translation"=6, "Back translation"=12, "Turning right"=0, "Turning left"=15, "Forward translation"=3, "Left translation"=9, "Gyro rotating"=16] ("Gait")
        # "左转90"
        n131 = Greater?(x=w290, y=3500 ("次数")) -> (0:w296:bool[])
        n132 = Or Array Elements(Boolean array=w296) -> (logical OR=w295:bool)
        n133 = call "步态方向转换 (子VI).vi"("速度"=30, "Gait"=w294) -> ("输出"=w293:dbl[])  [unwired: 9 in]
        n134 = Increment(x=w292) -> (x+1=w291:u16)
        n135 = Select(t=w291, s=w295, f=w292) -> (s? t:f=w298:u16)
      }
      frame 18 {
        w304 = i8 0 items=["Stop"=-1, "Right translation"=6, "Back translation"=12, "Turning right"=0, "Turning left"=15, "Forward translation"=3, "Left translation"=9, "Gyro rotating"=16] ("Gait")
        w322 = i8 9 items=["Stop"=-1, "Right translation"=6, "Back translation"=12, "Turning right"=0, "Turning left"=15, "Forward translation"=3, "Left translation"=9, "Gyro rotating"=16] ("Gait")
        # "左平移到物品架"
        n136 = Index Array(array=w323, index #1=1 ("索引")) -> (element #1=w303:dbl, element #2=w302:dbl)  [unwired: 1 in]
        n137 = Add(x=w303, y=w302) -> (x+y=w308:dbl)
        n138 = Divide(x=w308, y=2.0) -> (x/y=w306:dbl)
        n139 = Subtract(x=w306, y=100000.0) -> (x-y=w321:dbl)
        n140 = Subtract(x=w303, y=w302) -> (x-y=w305:dbl)
        n141 = Divide(x=w321, y=2.0 ("x")) -> (x/y=w311:dbl)
        n142 = call "步态方向转换 (子VI).vi"("速度"=w311, "Gait"=w322) -> ("输出"=w301:dbl[])  [unwired: 9 in]
        n143 = Increment(x=w325) -> (x+1=w324:u16)
        n144 = call "步态方向转换 (子VI).vi"("速度"=w305, "Gait"=w304) -> ("输出"=w300:dbl[])  [unwired: 9 in]
        n145 = Add(x=w301, y=w300) -> (x+y=w299:dbl[])
        n146 = call "PD.vi"("ENC"=w319, "SET"=w299) -> ("output"=w313:dbl[])  [unwired: 9 in]
        n147 = Less?(x=w313, y=0.5) -> (x < y?=w317:bool[])
        n148 = And Array Elements(Boolean array=w317) -> (logical AND=w316:bool)
        n149 = call "稳定T？.vi"("次数(100)"=30.0, "Reset"=w312, "输入"=w316) -> ("TT？"=w314:bool)  [unwired: 8 in]
        n150 = Select(t=w324, s=w314, f=w325) -> (s? t:f=w327:u16)
      }
      frame 19 {
        w339 = i8 12 items=["Stop"=-1, "Right translation"=6, "Back translation"=12, "Turning right"=0, "Turning left"=15, "Forward translation"=3, "Left translation"=9, "Gyro rotating"=16] ("Gait")
        # "货物架后扫线"
        n151 = Increment(x=w332) -> (x+1=w330:u16)
        n152 = call "rise.vi"("TF"=w329) -> ("UP?"=w328:bool)  [unwired: 10 in]
        n153 = call "计数器.vi"("Reset"=w331, "次数"=w330, "UP?"=w328) -> ("大于?"=w333:bool)  [unwired: 8 in]
        n154 = call "步态方向转换 (子VI).vi"("速度"=15, "Gait"=w339) -> ("输出"=w337:dbl[])  [unwired: 9 in]
        n155 = Increment(x=w336) -> (x+1=w335:u16)
        n156 = Select(t=w335, s=w333, f=w336) -> (s? t:f=w334:u16)
      }
      frame 20 {
        # "测场3"
        # "起夹手"
        n157 = Index Array(array=w341, index=5 ("索引")) -> (element=w344:i32)
        n158 = Less Or Equal?(x=w344, y=13000) -> (x <= y?=w342:bool)
        n159 = Increment(x=w347) -> (x+1=w340:u16)
        n160 = Select(t=w340, s=w342, f=w347) -> (s? t:f=w348:u16)
      }
      frame 21 {
        w356 = i8 15 items=["Stop"=-1, "Right translation"=6, "Back translation"=12, "Turning right"=0, "Turning left"=15, "Forward translation"=3, "Left translation"=9, "Gyro rotating"=16] ("Gait")
        # "左转90"
        n161 = Greater?(x=w352, y=3500 ("次数")) -> (0:w358:bool[])
        n162 = Or Array Elements(Boolean array=w358) -> (logical OR=w357:bool)
        n163 = call "步态方向转换 (子VI).vi"("速度"=30, "Gait"=w356) -> ("输出"=w355:dbl[])  [unwired: 9 in]
        n164 = Increment(x=w354) -> (x+1=w353:u16)
        n165 = Select(t=w353, s=w357, f=w354) -> (s? t:f=w360:u16)
      }
      frame 22 {
        w375 = i8 3 items=["Stop"=-1, "Right translation"=6, "Back translation"=12, "Turning right"=0, "Turning left"=15, "Forward translation"=3, "Left translation"=9, "Gyro rotating"=16] ("Gait")
        # "物品架前对正"
        n166 = Index Array(array=w376) -> (element=w361:dbl)  [unwired: 1 in]
        n167 = Subtract(x=w361, y=95000.0) -> (x-y=w374:dbl)
        n168 = Divide(x=w374, y=2.0 ("x")) -> (x/y=w363:dbl)
        n169 = Increment(x=w378) -> (x+1=w377:u16)
        n170 = call "步态方向转换 (子VI).vi"("速度"=w363, "Gait"=w375) -> ("输出"=w373:dbl[])  [unwired: 9 in]
        n171 = call "PD.vi"("ENC"=w371, "SET"=w373) -> ("output"=w365:dbl[])  [unwired: 9 in]
        n172 = Less?(x=w365, y=0.5) -> (x < y?=w369:bool[])
        n173 = And Array Elements(Boolean array=w369) -> (logical AND=w368:bool)
        n174 = call "稳定T？.vi"("次数(100)"=30.0, "Reset"=w364, "输入"=w368) -> ("TT？"=w366:bool)  [unwired: 8 in]
        n175 = Select(t=w377, s=w366, f=w378) -> (s? t:f=w380:u16)
      }
      frame 23 {
        w387 = i8 6 items=["Stop"=-1, "Right translation"=6, "Back translation"=12, "Turning right"=0, "Turning left"=15, "Forward translation"=3, "Left translation"=9, "Gyro rotating"=16] ("Gait")
        # "货物架右扫线"
        n176 = call "步态方向转换 (子VI).vi"("速度"=15, "Gait"=w387) -> ("输出"=w385:dbl[])  [unwired: 9 in]
        n177 = Increment(x=w384) -> (x+1=w383:u16)
        n178 = Select(t=w383, s=w381, f=w384) -> (s? t:f=w382:u16)
      }
      frame 24 {
        # "下抓手"
        n179 = Index Array(array=w389, index=5 ("索引")) -> (element=w392:i32)
        n180 = Greater Or Equal?(x=w392, y=14600) -> (x >= y?=w390:bool)
        n181 = Increment(x=w395) -> (x+1=w388:u16)
        n182 = Select(t=w388, s=w390, f=w395) -> (s? t:f=w396:u16)
      }
      frame 25 {
        # "抓取"
        n183 = Index Array(array=w399, index=4 ("索引")) -> (element=w402:i32)
        n184 = Less Or Equal?(x=w402, y=700) -> (x <= y?=w400:bool)
        n185 = Increment(x=w405) -> (x+1=w398:u16)
        n186 = Select(t=w398, s=w400, f=w405) -> (s? t:f=w406:u16)
      }
      frame 26 {
        # "抬升"
        n187 = Index Array(array=w409, index=5 ("索引")) -> (element=w412:i32)
        n188 = Less Or Equal?(x=w412, y=11800) -> (x <= y?=w410:bool)
        n189 = Increment(x=w415) -> (x+1=w408:u16)
        n190 = Select(t=w408, s=w410, f=w415) -> (s? t:f=w416:u16)
      }
      frame 27 {
        w424 = i8 15 items=["Stop"=-1, "Right translation"=6, "Back translation"=12, "Turning right"=0, "Turning left"=15, "Forward translation"=3, "Left translation"=9, "Gyro rotating"=16] ("Gait")
        # "左转90"
        n191 = Greater?(x=w419, y=3500 ("次数")) -> (0:w426:bool[])
        n192 = Or Array Elements(Boolean array=w426) -> (logical OR=w425:bool)
        n193 = call "步态方向转换 (子VI).vi"("速度"=w423, "Gait"=w424) -> ("输出"=w422:dbl[])  [unwired: 9 in]
        n194 = Increment(x=w421) -> (x+1=w420:u16)
        n195 = Select(t=w420, s=w425, f=w421) -> (s? t:f=w428:u16)
      }
      frame 28 {
        w434 = i8 0 items=["Stop"=-1, "Right translation"=6, "Back translation"=12, "Turning right"=0, "Turning left"=15, "Forward translation"=3, "Left translation"=9, "Gyro rotating"=16] ("Gait")
        w452 = i8 9 items=["Stop"=-1, "Right translation"=6, "Back translation"=12, "Turning right"=0, "Turning left"=15, "Forward translation"=3, "Left translation"=9, "Gyro rotating"=16] ("Gait")
        # "左平移到组装架"
        n196 = Index Array(array=w453, index #1=1 ("索引")) -> (element #1=w433:dbl, element #2=w432:dbl)  [unwired: 1 in]
        n197 = Add(x=w433, y=w432) -> (x+y=w438:dbl)
        n198 = Divide(x=w438, y=2.0) -> (x/y=w436:dbl)
        n199 = Subtract(x=w436, y=95000.0) -> (x-y=w451:dbl)
        n200 = Subtract(x=w433, y=w432) -> (x-y=w435:dbl)
        n201 = Divide(x=w451, y=2.0 ("x")) -> (x/y=w441:dbl)
        n202 = call "步态方向转换 (子VI).vi"("速度"=w441, "Gait"=w452) -> ("输出"=w431:dbl[])  [unwired: 9 in]
        n203 = Increment(x=w455) -> (x+1=w454:u16)
        n204 = call "步态方向转换 (子VI).vi"("速度"=w435, "Gait"=w434) -> ("输出"=w430:dbl[])  [unwired: 9 in]
        n205 = Add(x=w431, y=w430) -> (x+y=w429:dbl[])
        n206 = call "PD.vi"("ENC"=w449, "SET"=w429) -> ("output"=w443:dbl[])  [unwired: 9 in]
        n207 = Less?(x=w443, y=0.5) -> (x < y?=w447:bool[])
        n208 = And Array Elements(Boolean array=w447) -> (logical AND=w446:bool)
        n209 = call "稳定T？.vi"("次数(100)"=30.0, "Reset"=w442, "输入"=w446) -> ("TT？"=w444:bool)  [unwired: 8 in]
        n210 = Select(t=w454, s=w444, f=w455) -> (s? t:f=w457:u16)
      }
      frame 29 {
        w464 = i8 12 items=["Stop"=-1, "Right translation"=6, "Back translation"=12, "Turning right"=0, "Turning left"=15, "Forward translation"=3, "Left translation"=9, "Gyro rotating"=16] ("Gait")
        # "组装台后扫线"
        n211 = call "步态方向转换 (子VI).vi"("速度"=15, "Gait"=w464) -> ("输出"=w462:dbl[])  [unwired: 9 in]
        n212 = Increment(x=w461) -> (x+1=w460:u16)
        n213 = Select(t=w460, s=w458, f=w461) -> (s? t:f=w459:u16)
      }
      frame 30 {
        w471 = i8 15 items=["Stop"=-1, "Right translation"=6, "Back translation"=12, "Turning right"=0, "Turning left"=15, "Forward translation"=3, "Left translation"=9, "Gyro rotating"=16] ("Gait")
        # "左转90"
        n214 = Greater?(x=w467, y=3500 ("次数")) -> (0:w473:bool[])
        n215 = Or Array Elements(Boolean array=w473) -> (logical OR=w472:bool)
        n216 = call "步态方向转换 (子VI).vi"("速度"=30, "Gait"=w471) -> ("输出"=w470:dbl[])  [unwired: 9 in]
        n217 = Increment(x=w469) -> (x+1=w468:u16)
        n218 = Select(t=w468, s=w472, f=w469) -> (s? t:f=w475:u16)
      }
      frame 31 {
        w488 = i8 3 items=["Stop"=-1, "Right translation"=6, "Back translation"=12, "Turning right"=0, "Turning left"=15, "Forward translation"=3, "Left translation"=9, "Gyro rotating"=16] ("Gait")
        # "组装台前对正"
        n219 = Index Array(array=w489) -> (element=w477:dbl)  [unwired: 1 in]
        n220 = Subtract(x=w477, y=93000.0) -> (x-y=w476:dbl)
        n221 = Increment(x=w491) -> (x+1=w490:u16)
        n222 = call "步态方向转换 (子VI).vi"("速度"=w476, "Gait"=w488) -> ("输出"=w487:dbl[])  [unwired: 9 in]
        n223 = call "PD.vi"("ENC"=w485, "SET"=w487) -> ("output"=w479:dbl[])  [unwired: 9 in]
        n224 = Less?(x=w479, y=0.5) -> (x < y?=w483:bool[])
        n225 = And Array Elements(Boolean array=w483) -> (logical AND=w482:bool)
        n226 = call "稳定T？.vi"("次数(100)"=30.0, "Reset"=w478, "输入"=w482) -> ("TT？"=w480:bool)  [unwired: 8 in]
        n227 = Select(t=w490, s=w480, f=w491) -> (s? t:f=w493:u16)
      }
      frame 32 {
        w500 = i8 6 items=["Stop"=-1, "Right translation"=6, "Back translation"=12, "Turning right"=0, "Turning left"=15, "Forward translation"=3, "Left translation"=9, "Gyro rotating"=16] ("Gait")
        # "组装台右扫线"
        n228 = call "步态方向转换 (子VI).vi"("速度"=15, "Gait"=w500) -> ("输出"=w498:dbl[])  [unwired: 9 in]
        n229 = Increment(x=w497) -> (x+1=w496:u16)
        n230 = Select(t=w496, s=w494, f=w497) -> (s? t:f=w495:u16)
      }
      frame 33 {
        # "730"
        # "松夹手"
        n231 = Index Array(array=w502, index=4 ("索引")) -> (element=w505:i32)
        n232 = Greater Or Equal?(x=w505, y=800) -> (x >= y?=w503:bool)
        n233 = Increment(x=w508) -> (x+1=w501:u16)
        n234 = Select(t=w501, s=w503, f=w508) -> (s? t:f=w509:u16)
      }
      frame 34 {
        w520 = i8 12 items=["Stop"=-1, "Right translation"=6, "Back translation"=12, "Turning right"=0, "Turning left"=15, "Forward translation"=3, "Left translation"=9, "Gyro rotating"=16] ("Gait")
        # "测场8"
        # "组装架后退"
        n235 = Greater?(x=w512, y=2000) -> (0:w513:bool[])
        n236 = Or Array Elements(Boolean array=w513) -> (logical OR=w511:bool)
        n237 = Increment(x=w516) -> (x+1=w515:u16)
        n238 = call "步态方向转换 (子VI).vi"("速度"=15, "Gait"=w520) -> ("输出"=w518:dbl[])  [unwired: 9 in]
        n239 = Select(t=w515, s=w511, f=w516) -> (s? t:f=w517:u16)
      }
      frame 35 {
        # "测场1"
        # "组装架下夹手"
        n240 = Index Array(array=w523, index=5 ("索引")) -> (element=w526:i32)
        n241 = Greater Or Equal?(x=w526, y=15100) -> (x >= y?=w524:bool)
        n242 = Increment(x=w529) -> (x+1=w522:u16)
        n243 = Select(t=w522, s=w524, f=w529) -> (s? t:f=w530:u16)
      }
      frame 36 {
        w541 = i8 3 items=["Stop"=-1, "Right translation"=6, "Back translation"=12, "Turning right"=0, "Turning left"=15, "Forward translation"=3, "Left translation"=9, "Gyro rotating"=16] ("Gait")
        # "组装架前进插托盘"
        n244 = Greater?(x=w536, y=2000) -> (0:w537:bool[])
        n245 = Or Array Elements(Boolean array=w537) -> (logical OR=w535:bool)
        n246 = call "步态方向转换 (子VI).vi"("速度"=15, "Gait"=w541) -> ("输出"=w539:dbl[])  [unwired: 9 in]
        n247 = Increment(x=w533) -> (x+1=w534:u16)
        n248 = Select(t=w534, s=w535, f=w533) -> (s? t:f=w532:u16)
      }
      frame 37 {
        # "起托盘"
        n249 = Index Array(array=w543, index=5 ("索引")) -> (element=w546:i32)
        n250 = Less Or Equal?(x=w546, y=8000) -> (x <= y?=w544:bool)
        n251 = Increment(x=w549) -> (x+1=w542:u16)
        n252 = Select(t=w542, s=w544, f=w549) -> (s? t:f=w550:u16)
      }
      frame 38 {
        w558 = i8 0 items=["Stop"=-1, "Right translation"=6, "Back translation"=12, "Turning right"=0, "Turning left"=15, "Forward translation"=3, "Left translation"=9, "Gyro rotating"=16] ("Gait")
        # "右转90"
        n253 = Greater?(x=w554, y=3550 ("次数")) -> (0:w560:bool[])
        n254 = Or Array Elements(Boolean array=w560) -> (logical OR=w559:bool)
        n255 = call "步态方向转换 (子VI).vi"("速度"=20, "Gait"=w558) -> ("输出"=w557:dbl[])  [unwired: 9 in]
        n256 = Increment(x=w556) -> (x+1=w555:u16)
        n257 = Select(t=w555, s=w559, f=w556) -> (s? t:f=w562:u16)
      }
      frame 39 {
        w571 = i8 3 items=["Stop"=-1, "Right translation"=6, "Back translation"=12, "Turning right"=0, "Turning left"=15, "Forward translation"=3, "Left translation"=9, "Gyro rotating"=16] ("Gait")
        # "前进到交付区"
        n258 = Greater?(x=w570, y=13000) -> (0:w567:bool[])
        n259 = Or Array Elements(Boolean array=w567) -> (logical OR=w564:bool)
        n260 = Increment(x=w565) -> (x+1=w566:u16)
        n261 = call "步态方向转换 (子VI).vi"("速度"=30, "Gait"=w571) -> ("输出"=w572:dbl[])  [unwired: 9 in]
        n262 = Select(t=w566, s=w564, f=w565) -> (s? t:f=w568:u16)
      }
      frame 40 {
        # "对正"
        n263 = feedback-in #7(w585) -> ()
        n264 = feedback #7() -> (w584:i32[])  [unwired: 1 in]
        n265 = Subtract(x=w585, y=w584) -> (x-y=w583:i32[])
        n266 = call "超声波对正(子VI).vi"("LFT"=45000.0, "FWD"=100000.0, "超声波"=w590) -> ("数组输出"=w589:dbl[])  [unwired: 8 in]
        n267 = Increment(x=w588) -> (x+1=w573:u16)
        n268 = disable-structure shown="禁用" {
          disable-tunnel: w589 -> [w593 w594]
          disable-tunnel: [w591 w594] -> w586
          frame Disabled {
            n269 = call "限速.vi"("最大值"=60.0, "输入"=w593) -> ("数组"=w591:dbl[])  [unwired: 9 in]
          }
          frame Enabled {
          }
        }
        n270 = call "PD.vi"("ENC"=w583, "SET"=w586) -> ("output"=w582:dbl[])  [unwired: 9 in]
        n271 = Less?(x=w582, y=0.5) -> (x < y?=w580:bool[])
        n272 = And Array Elements(Boolean array=w580) -> (logical AND=w579:bool)
        n273 = call "稳定T？.vi"("次数(100)"=100.0, "Reset"=w577, "输入"=w579) -> ("TT？"=w578:bool)  [unwired: 8 in]
        n274 = Select(t=w573, s=w578, f=w588) -> (s? t:f=w587:u16)
      }
      frame 41 {
        w605 = i8 6 items=["Stop"=-1, "Right translation"=6, "Back translation"=12, "Turning right"=0, "Turning left"=15, "Forward translation"=3, "Left translation"=9, "Gyro rotating"=16] ("Gait")
        # "交付区右扫线"
        n275 = call "rise.vi"("TF"=w596) -> ("UP?"=w595:bool)  [unwired: 10 in]
        n276 = call "计数器.vi"("Reset"=w598, "次数"=w597, "UP?"=w595) -> ("大于?"=w599:bool)  [unwired: 8 in]
        n277 = call "步态方向转换 (子VI).vi"("速度"=15, "Gait"=w605) -> ("输出"=w603:dbl[])  [unwired: 9 in]
        n278 = Increment(x=w602) -> (x+1=w601:u16)
        n279 = Select(t=w601, s=w599, f=w602) -> (s? t:f=w600:u16)
      }
      frame 42 {
        # "下抓手"
        n280 = Index Array(array=w608, index=5 ("索引")) -> (element=w611:i32)
        n281 = Greater Or Equal?(x=w611, y=13200) -> (x >= y?=w609:bool)
        n282 = Increment(x=w614) -> (x+1=w607:u16)
        n283 = Select(t=w607, s=w609, f=w614) -> (s? t:f=w615:u16)
      }
      frame 43 {
        w626 = i8 12 items=["Stop"=-1, "Right translation"=6, "Back translation"=12, "Turning right"=0, "Turning left"=15, "Forward translation"=3, "Left translation"=9, "Gyro rotating"=16] ("Gait")
        # "测场8"
        # "返回区后退"
        n284 = Greater?(x=w618, y=10000) -> (0:w619:bool[])
        n285 = Or Array Elements(Boolean array=w619) -> (logical OR=w617:bool)
        n286 = Increment(x=w622) -> (x+1=w621:u16)
        n287 = call "步态方向转换 (子VI).vi"("速度"=30, "Gait"=w626) -> ("输出"=w624:dbl[])  [unwired: 9 in]
        n288 = Select(t=w621, s=w617, f=w622) -> (s? t:f=w623:u16)
      }
      frame 45 {
        w631 = i8 3 items=["Stop"=-1, "Right translation"=6, "Back translation"=12, "Turning right"=0, "Turning left"=15, "Forward translation"=3, "Left translation"=9, "Gyro rotating"=16] ("Gait")
        w630 = 30 ("速度")
        w639 = i8 9 items=["Stop"=-1, "Right translation"=6, "Back translation"=12, "Turning right"=0, "Turning left"=15, "Forward translation"=3, "Left translation"=9, "Gyro rotating"=16] ("Gait")
        # "测场8"
        # "返回区左前平移"
        n289 = Greater?(x=w633, y=2000) -> (0:w634:bool[])
        n290 = Or Array Elements(Boolean array=w634) -> (logical OR=w632:bool)
        n291 = Increment(x=w637) -> (x+1=w636:u16)
        n292 = call "步态方向转换 (子VI).vi"("速度"=w630, "Gait"=w631) -> ("输出"=w628:dbl[])  [unwired: 9 in]
        n293 = call "步态方向转换 (子VI).vi"("速度"=w630, "Gait"=w639) -> ("输出"=w629:dbl[])  [unwired: 9 in]
        n294 = Add(x=w628, y=w629) -> (x+y=w627:dbl[])
        n295 = Select(t=w636, s=w632, f=w637) -> (s? t:f=w638:u16)
      }
      frame 44 {
        w646 = i8 15 items=["Stop"=-1, "Right translation"=6, "Back translation"=12, "Turning right"=0, "Turning left"=15, "Forward translation"=3, "Left translation"=9, "Gyro rotating"=16] ("Gait")
        # "转身"
        n296 = Greater?(x=w641, y=7000 ("次数")) -> (0:w648:bool[])
        n297 = Or Array Elements(Boolean array=w648) -> (logical OR=w647:bool)
        n298 = call "步态方向转换 (子VI).vi"("速度"=w645, "Gait"=w646) -> ("输出"=w644:dbl[])  [unwired: 9 in]
        n299 = Increment(x=w643) -> (x+1=w642:u16)
        n300 = Select(t=w642, s=w647, f=w643) -> (s? t:f=w650:u16)
      }
      frame 46 {
        # "对正"
        n301 = feedback-in #8(w663) -> ()
        n302 = feedback #8() -> (w662:i32[])  [unwired: 1 in]
        n303 = Subtract(x=w663, y=w662) -> (x-y=w661:i32[])
        n304 = call "超声波对正(子VI).vi"("LFT"=100000.0, "FWD"=100000.0, "超声波"=w668) -> ("数组输出"=w667:dbl[])  [unwired: 8 in]
        n305 = disable-structure shown="禁用" {
          disable-tunnel: w667 -> [w671 w672]
          disable-tunnel: [w669 w672] -> w664
          frame Disabled {
            n306 = call "限速.vi"("最大值"=60.0, "输入"=w671) -> ("数组"=w669:dbl[])  [unwired: 9 in]
          }
          frame Enabled {
          }
        }
        n307 = call "PD.vi"("ENC"=w661, "SET"=w664) -> ("output"=w660:dbl[])  [unwired: 9 in]
        n308 = Less?(x=w660, y=0.5) -> (x < y?=w658:bool[])
        n309 = And Array Elements(Boolean array=w658) -> (logical AND=w657:bool)
        n310 = call "稳定T？.vi"("次数(100)"=100.0, "Reset"=w655, "输入"=w657) -> ("TT？"=w656:bool)  [unwired: 8 in]
        n311 = Select(t=u16 4, s=w656, f=w666) -> (s? t:f=w665:u16)
      }
      frame 50 {
        n312 = Index Array(array=w673, index=4 ("索引")) -> (element=w676:i32)
        n313 = Less Or Equal?(x=w676, y=50) -> (x <= y?=w674:bool)
        n314 = Increment(x=w679) -> (x+1=w680:u16)
        n315 = Select(t=w680, s=w674, f=w679) -> (s? t:f=w681:u16)
      }
      frame 51 {
        n316 = Index Array(array=w685, index=5 ("索引")) -> (element=w688:i32)
        n317 = Less Or Equal?(x=w688, y=100) -> (x <= y?=w686:bool)
        n318 = Increment(x=w691) -> ()  [unwired: 1 out]
        n319 = Select(t=u16 0, s=w686, f=w691) -> (s? t:f=w692:u16)
      }
      frame 52 {
        w699 = i8 12 items=["Stop"=-1, "Right translation"=6, "Back translation"=12, "Turning right"=0, "Turning left"=15, "Forward translation"=3, "Left translation"=9, "Gyro rotating"=16] ("Gait")
        n320 = Greater?(x=w696, y=8000 ("长度 2")) -> (0:w697:bool[])
        n321 = Or Array Elements(Boolean array=w697) -> (logical OR=w695:bool)
        n322 = call "步态方向转换 (子VI).vi"("速度"=w694, "Gait"=w699) -> ("输出"=w700:dbl[])  [unwired: 9 in]
        n323 = Select(t=u16 0, s=w695, f=w702) -> (s? t:f=w703:u16)
      }
      frame 96 {
        # "抓"
        n324 = Index Array(array=w704, index=4 ("索引")) -> (element=w707:i32)
        n325 = Less Or Equal?(x=w707, y=700) -> (x <= y?=w705:bool)
        n326 = Increment(x=w710) -> (x+1=w711:u16)
        n327 = Select(t=w711, s=w705, f=w710) -> (s? t:f=w712:u16)
      }
      frame 99 {
        # "货物类型判断"
        n328 = Array Max & Min(array=dbl[] [] ("数组")) -> (max value=w727:dbl, max index (indices)=w722:i32)  [unwired: 2 out]
        n329 = Greater Or Equal?(x=w727, y=50000.0 ("大小阈值")) -> (x >= y?=w728:bool)
        n330 = Select(t=1.0, s=w728, f=3.0) -> (s? t:f=w723:dbl)
        n331 = feedback #9() -> (w717:dbl)  [unwired: 1 in]
        n332 = Add(x=w723, y=w722) -> (x+y=w716:dbl)
        n333 = feedback-in #9(w716) -> ()
        n334 = Not Equal?(x=w716, y=w717) -> (x != y?=w715:bool)
        n335 = Increment(x=w718) -> (x+1=w719:u16)
        n336 = Select(t=w719, s=w715, f=w718) -> (s? t:f=w720:u16)
      }
      frame 100 {
        # "停止"
      }
    }
    n337 = Select(t=FALSE, s=w49, f=w52) -> (s? t:f=w51:bool)
    n338 = call "缓起(子VI).vi"("缓起清零"=w51, "输入"=w71) -> ("输出"=w73:i32[])  [unwired: 9 in]
    n339 = Not(x=w69) -> (.not. x?=w68:bool)
    n340 = Select(t=u16 0, s="Reset to gait 0", f=w55) -> (s? t:f=w46:u16)
    n341 = call "PID.vi"("继电器"=w68, "SET"=w73, "ENC"=w62) -> ("DIR"=w77:bool[], "PWM"=w78:dbl[])  [unwired: 7 in]
    n342 = Select(t=u16 50, s="Reset", f=w46) -> (s? t:f=w45:u16)
    n343 = call "DIR RT.vi"("DIR"=w77, "Custom FPGA Reference Out"=w60) -> ()  [unwired: 8 in, 2 out]
    n344 = call "PWM RT总.vi"("PWM"=w78, "Custom FPGA Reference Out"=w60) -> ()  [unwired: 8 in, 2 out]
    n345 = Select(t=u16 100 ("f"), s="停止", f=w45) -> (s? t:f=w58:u16)
    n346 = node-c288() -> ()  [unwired: 1 in, 1 out]
    n347 = local write "停止 2"(w44) -> ()
    "当前步态" <- w33
  }
  n348 = while {
    tunnel: w18 -> [w751]
    tunnel: w8 -> [w744]
    tunnel: w7 -> [w743]
    tunnel: w20 -> [w753]
    tunnel: [w752] -> w19
    tunnel: w6 -> [w740]
    tunnel: [w739] -> w5
    stop <- "停止 2" stop-if-true
    # "图像处理"
    n349 = Build Array(w744, w743) -> (w750:T2[])
    n350 = call <vilib>:"IMAQdx Grab2.vi"("Image In"=w751, "Session In"=w753) -> ("Image Out"=w745:T2, "Session Out"=w752:T1)  [unwired: 6 in, 2 out]
    n351 = for {
      tunnel: cluster{"Lower value":i32, "Upper value":i32}[] [{"Lower value"=220, "Upper value"=255}, {"Lower value"=0, "Upper value"=100}] -> [w781] mode=indexing
      tunnel: cluster{"Lower value":i32, "Upper value":i32}[] [{"Lower value"=0, "Upper value"=106}, {"Lower value"=75, "Upper value"=200}] -> [w780] mode=indexing
      tunnel: cluster{"Lower value":i32, "Upper value":i32}[] [{"Lower value"=5, "Upper value"=97}, {"Lower value"=170, "Upper value"=255}] -> [w779] mode=indexing
      tunnel: [w761] -> w746 mode=indexing
      tunnel: [w760] -> w742 mode=indexing
      tunnel: w745 -> [w754]
      tunnel: w750 -> [w759] mode=indexing
      tunnel: w740 -> [w758]
      tunnel: [w757] -> w739
      tunnel: [w755] -> _ mode=indexing
      tunnel: [w754] -> _ mode=indexing
      w767 = i32[] [] items=["Center of Mass X", "Center of Mass Y", "First Pixel X", "First Pixel Y", "Bounding Rect Left", "Bounding Rect Top", "Bounding Rect Right", "Bounding Rect Bottom", "Max Feret Diameter Start X", "Max Feret Diameter Start Y", "Max Feret Diameter End X", "Max Feret Diameter End Y", "Max Horiz. Segment Length Left", "Max Horiz. Segment Length Right", "Max Horiz. Segment Length Row", "-", "Bounding Rect Width", "Bounding Rect Height", "Bounding Rect Diagonal", "Perimeter", "Convex Hull Perimeter", "Holes' Perimeter", "Max Feret Diameter", "Equivalent Ellipse Major Axis", "Equivalent Ellipse Minor Axis", "Equivalent Ellipse Minor Axis (Feret)", "Equivalent Rect Long Side", "Equivalent Rect Short Side", "Equivalent Rect Diagonal", "Equivalent Rect Short Side (Feret)", "Average Horiz. Segment Length", "Average Vert. Segment Length", "Hydraulic Radius", "Waddel Disk Diameter", "-", "Area", "Holes' Area", "Particle & Holes' Area", "Convex Hull Area", "Image Area", "-", "Number of Holes", "Number of Horiz. Segments", "Number of Vert. Segments", "-", "Orientation", "Max Feret Diameter Orientation", "-", "% Area/Image Area", "% Area/(Particle & Holes' Area)", "Ratio of Equivalent Ellipse Axes", "Ratio of Equivalent Rect Sides", "-", "Elongation Factor", "Compactness Factor", "Heywood Circularity Factor", "Type Factor", "-", "Sum X", "Sum Y", "Sum XX", "Sum XY", "Sum YY", "Sum XXX", "Sum XXY", "Sum XYY", "Sum YYY", "-", "Moment of Inertia XX", "Moment of Inertia XY", "Moment of Inertia YY", "Moment of Inertia XXX", "Moment of Inertia XXY", "Moment of Inertia XYY", "Moment of Inertia YYY", "Norm. Moment of Inertia XX", "Norm. Moment of Inertia XY", "Norm. Moment of Inertia YY", "Norm. Moment of Inertia XXX", "Norm. Moment of Inertia XXY", "Norm. Moment of Inertia XYY", "Norm. Moment of Inertia YYY", "Hu Moment 1", "Hu Moment 2", "Hu Moment 3", "Hu Moment 4", "Hu Moment 5", "Hu Moment 6", "Hu Moment 7"] ("Real-World Measurements")
      w768 = i32[] [35] items=["Center of Mass X", "Center of Mass Y", "First Pixel X", "First Pixel Y", "Bounding Rect Left", "Bounding Rect Top", "Bounding Rect Right", "Bounding Rect Bottom", "Max Feret Diameter Start X", "Max Feret Diameter Start Y", "Max Feret Diameter End X", "Max Feret Diameter End Y", "Max Horiz. Segment Length Left", "Max Horiz. Segment Length Right", "Max Horiz. Segment Length Row", "-", "Bounding Rect Width", "Bounding Rect Height", "Bounding Rect Diagonal", "Perimeter", "Convex Hull Perimeter", "Holes' Perimeter", "Max Feret Diameter", "Equivalent Ellipse Major Axis", "Equivalent Ellipse Minor Axis", "Equivalent Ellipse Minor Axis (Feret)", "Equivalent Rect Long Side", "Equivalent Rect Short Side", "Equivalent Rect Diagonal", "Equivalent Rect Short Side (Feret)", "Average Horiz. Segment Length", "Average Vert. Segment Length", "Hydraulic Radius", "Waddel Disk Diameter", "-", "Area", "Holes' Area", "Particle & Holes' Area", "Convex Hull Area", "Image Area", "-", "Number of Holes", "Number of Horiz. Segments", "Number of Vert. Segments", "-", "Orientation", "Max Feret Diameter Orientation", "-", "% Area/Image Area", "% Area/(Particle & Holes' Area)", "Ratio of Equivalent Ellipse Axes", "Ratio of Equivalent Rect Sides", "-", "Elongation Factor", "Compactness Factor", "Heywood Circularity Factor", "Type Factor", "-", "Sum X", "Sum Y", "Sum XX", "Sum XY", "Sum YY", "Sum XXX", "Sum XXY", "Sum XYY", "Sum YYY", "-", "Moment of Inertia XX", "Moment of Inertia XY", "Moment of Inertia YY", "Moment of Inertia XXX", "Moment of Inertia XXY", "Moment of Inertia XYY", "Moment of Inertia YYY", "Norm. Moment of Inertia XX", "Norm. Moment of Inertia XY", "Norm. Moment of Inertia YY", "Norm. Moment of Inertia XXX", "Norm. Moment of Inertia XXY", "Norm. Moment of Inertia XYY", "Norm. Moment of Inertia YYY", "Hu Moment 1", "Hu Moment 2", "Hu Moment 3", "Hu Moment 4", "Hu Moment 5", "Hu Moment 6", "Hu Moment 7"] ("Pixel Measurements")
      w765 = TRUE ("Connectivity 4/8 (8)")
      w782 = u16 0 items=["RGB", "HSL", "HSV", "HSI"] ("Color Mode")
      n352 = call "IMAQ ColorThreshold"("Blue or Luma or Val or Inten Range"=w779, "Replace Value"=1, "Green or Sat Range"=w780, "Color Mode"=w782, "error in (no error)"=w758, "Red or Hue Range"=w781, "Image Dst"=w759, "Image Src"=w754) -> ("error out"=w778:errorcluster, "Image Dst Out"=w773:T2)  [unwired: 2 out]
      n353 = call "IMAQ RemoveParticle"("Connectivity 4/8 (8)"=TRUE, "Low Pass/High Pass (Low)"=FALSE, "Square/Hexa (Square)"=FALSE, "error in (no error)"=w778, "Number of Erosion"=5, "Image Src"=w773) -> ("error out"=w772:errorcluster, "Image Dst Out"=w770:T2)  [unwired: 1 in, 3 out]
      n354 = call "IMAQ FillHole"("error in (no error)"=w772, "Image Src"=w770, "Connectivity 4/8 (8)"=TRUE) -> ("error out"=w769:errorcluster, "Image Dst Out"=w766:T2)  [unwired: 1 in, 2 out]
      n355 = call "IMAQ Particle Analysis"("Connectivity 4/8 (8)"=w765, "error in (no error)"=w769, "Real-World Measurements"=w767, "Pixel Measurements"=w768, "Image"=w766) -> ("error out"=w762:errorcluster, "Particle Measurements (Pixels)"=w760:dbl[][], "Image Out (duplicate)"=w764:T2)  [unwired: 4 out]
      n356 = Wait (ms)(milliseconds to wait=u32 5 ("等待时间（毫秒）")) -> ()  [unwired: 1 out]
      n357 = call <vilib>:"IVA Store Particles Results.vi"("error in (no error)"=w762, "Connectivity 4/8 (8)"=w765, "Step Name"="Particle Analysis 1", "Image in"=w764) -> ("error out"=w757:errorcluster, "Number of Particles"=w761:i32, "Image dup"=w755:T2)  [unwired: 5 out]
    }
    "数量" <- w746
    n358 = Reshape Array(w742, 2 ("维数大小")) -> (w737:dbl[])
    n359 = Greater?(x=w737, y=10000.0) -> (0:w735:bool[])
    n360 = Boolean Array To Number(Boolean array=w735) -> (number=→"货物类型":u32)
  }
  n361 = call <vilib>:"IMAQdx Close Camera.vi"("error in"=w5, "Session In"=w19) -> ("error out"=w17:errorcluster)  [unwired: 9 in]
  n362 = Not(x="保留图像？") -> (.not. x?=w3:bool)
  n363 = call "IMAQ Dispose"("All Images? (No)"=w3, "error in (no error)"=w17) -> ()  [unwired: 4 in, 1 out]
  n364 = node-c288(w29) -> (w27:errorcluster)
  n365 = xnode "关闭FPGA VI引用"("FPGA VI引用输入"=w21, "错误输入"=w27) -> ("错误输出"=w26:errorcluster)
  n366 = call <vilib>:"Reset myRIO.vi"("error in (no error)"=w26) -> ()  [unwired: 10 in, 1 out]
